vi "Set Package.vi"(7 "LabVIEW Web Service Request":refnum<class "Web Request.lvclass">) -> ()   [LabVIEW 2016]
uses:
  <vilib>/wsapi/Web Request.lvclass
  <vilib>/wsapi/class/subVIs/Write Single Session Variable.vi
  Libraries/WSsupport/WSsupport.lvlib
  Libraries/ServerErrors/ServerErrors.lvlib
panel:
  # "Use the Web Service Request input terminal to call the VIs on the Web Services palette. Do not remove it from the connector pane unless you don't need access to the palette."
  # "Each additional control wired to the connector pane will be available as an input in the URL. To include an indicator in terminal-mode output (the default setting), it must also be wired to the connector pane."
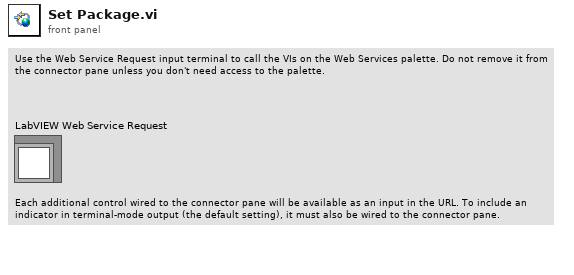
[diagram p1: front panel]
types:
  T1 = typedef "ServerErrors.lvlib/Error Message--cluster.ctl" = cluster{"HTTP Code":i32, "JSON Response":cluster{"error":string, "reason":string}}
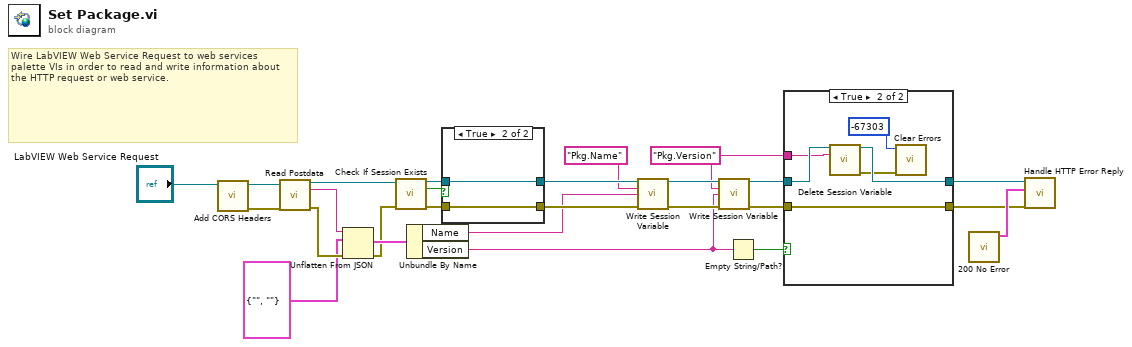
[diagram p0: block diagram]
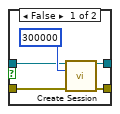
[diagram p3: hidden frame]
diagram:
  w2 = "Pkg.Version" ("key")
  # "Wire LabVIEW Web Service Request to web services palette VIs in order to read and write information about the HTTP request or web service."
  n1 = call "Add CORS Headers.vi"("LabVIEW Web Service Request"="LabVIEW Web Service Request") -> ("error out"=w24:errorcluster, "LabVIEW Web Service Request out"=w25:refnum<class "Web Request.lvclass">)  [unwired: 9 in]
  n2 = call <vilib>:"Read Postdata.vi"("LabVIEW Web Service Request"=w25, "error in (no error)"=w24) -> ("LabVIEW Web Service Request out"=w9:refnum<class "Web Request.lvclass">, "postdata"=w22:string, "error out"=w23:errorcluster)  [unwired: 11 in]
  n3 = Unflatten From JSON(JSON string=w22, type and defaults=cluster{"Name":string, "Version":string} {"Name"="", "Version"=""}, error in (no error)=w23) -> (value=w20:cluster{"Name":string, "Version":string}, error out=w19:errorcluster)  [unwired: 4 in]
  n4 = call <vilib>:"Check If Session Exists.vi"("LabVIEW Web Service Request"=w9, "error in (no error)"=w19) -> ("LabVIEW Web Service Request out"=w8:refnum<class "Web Request.lvclass">, "session exists?"=w7:bool, "error out"=w10:errorcluster)  [unwired: 11 in]
  n5 = Unbundle By Name(w20) -> ("Name"=w15:string, "Version"=w6:string)
  n6 = case shown="True" w7 {
    tunnel: [w30 w33] -> w18
    tunnel: [w29 w32] -> w17
    tunnel: w10 -> [w28 w32]
    tunnel: w8 -> [w27 w33]
    frame False {
      n7 = call <vilib>:"Create Session.vi"("LabVIEW Web Service Request"=w27, "timeout (60000 msec)"=u32 300000, "error in (no error)"=w28) -> ("LabVIEW Web Service Request out"=w30:refnum<class "Web Request.lvclass">, "error out"=w29:errorcluster)  [unwired: 10 in, 1 out]
    }
    frame True {
    }
  }
  n8 = call-poly <vilib>:"Write Session Variable.vi"("LabVIEW Web Service Request"=w18, "key"="Pkg.Name", "value"=w15, "error in (no error)"=w17) -> ("LabVIEW Web Service Request out"=w14:refnum<class "Web Request.lvclass">, "error out"=w13:errorcluster)  [unwired: 8 in, 2 out]
  n9 = call-poly <vilib>:"Write Session Variable.vi"("LabVIEW Web Service Request"=w14, "key"=w2, "value"=w6, "error in (no error)"=w13) -> ("LabVIEW Web Service Request out"=w4:refnum<class "Web Request.lvclass">, "error out"=w12:errorcluster)  [unwired: 8 in, 2 out]
  n10 = Empty String/Path?(string/path=w6) -> (empty?=w1:bool)
  n11 = case shown="True" w1 {
    tunnel: w12 -> [w34 w38]
    tunnel: [w34 w38] -> w5
    tunnel: w4 -> [w35 w41]
    tunnel: [w35 w40] -> w3
    tunnel: w2 -> [_ w39]
    frame False {
    }
    frame True {
      n12 = call <vilib>:"Delete Session Variable.vi"("LabVIEW Web Service Request"=w41, "key"=w39) -> ("LabVIEW Web Service Request out"=w40:refnum<class "Web Request.lvclass">, "error out"=w37:errorcluster)  [unwired: 12 in]
      n13 = call <vilib>:"Clear Errors.vi"("error in (no error)"=w37, "specific error code to clear (0: all)"=-67303) -> ()  [unwired: 4 in, 2 out]
    }
  }
  n14 = call "200 No Error.vi"() -> ("no error"=w11:T1)  [unwired: 11 in]
  n15 = call "Handle HTTP Error Reply.vi"("error in (no error)"=w5, "HTTP Status Code"=w11, "Web Request in"=w3) -> ()  [unwired: 8 in, 1 out]
